vi "probe_freq_sweep.vi"() -> ()   [LabVIEW 2017]
doc: "Use this template to build a simple state machine design pattern. Each state executes code and determines which state to transition to."
uses:
  controls/State.ctl
  <userlib>/niRF/niQuickSyn/Core/Properties/Ref Output/PropertyType.ctl
  <userlib>/niRF/niQuickSyn/Core/Properties/Reference Source/PropertyType.ctl
  <instrlib>/niRFSA/niRFSA.llb/niRFSA Acquisition Types.ctl
  <userlib>/niRF/niQuickSyn/Core/Properties/RF Output/PropertyType.ctl
  <userlib>/niRF/niQuickSyn/Core/Typedefs/Session Handle.ctl
  <userlib>/niRF/niQuickSyn/Core/QuickSyn.lvclass
  <vilib>/Utility/error.llb/DialogType.ctl
  <vilib>/Analysis/1siggen.llb/Ramp Pattern by Samples.vi
  <instrlib>/niRFSA/niRFSA.llb/niRFSA Configure Spectrum Frequency Start Stop.vi
  <instrlib>/niRFSA/niRFSA.llb/niRFSA Read Power Spectrum (DBL).vi
  <userlib>/niRF/niQuickSyn/QuickSyn API.lvlib
  <userlib>/niRF/niQuickSyn/Core/Properties/Ref Output/Ref Output.lvclass
  <userlib>/niRF/niQuickSyn/Core/Properties/Reference Source/Ref Source.lvclass
  <userlib>/niRF/niQuickSyn/Core/Properties/RF Output/RF Output.lvclass
  <vilib>/Analysis/NI_AALBase.lvlib
panel:
  in  "Averaging":i32=1000 min=1 max=3201 step=1
  out "error out":errorcluster
  out "QuickSyn Resource Name Out":refnum<visa-resource-name>
  out "RFSA Resource Name Out":refnum<k15>
  in  "error in (no error)":errorcluster
  in  "Folder":string="Test"
  in  "Resolution Bandwidth RFSA":dbl=100000.0 caption="Resolution Bandwidth (Hz)" min=1.0 max=25000000.0 step=1.0 format="%#_6p"
  in  "Reference Power RFSA":dbl=1.0 caption="Reference Level (dBm)" min=-25.0 max=13.0 step=0.1
  in  "Stop Frequncy RFSA":dbl=2000000000.0 caption="Stop Frequncy (Hz)" min=500000000.0 max=20000000000.0 format="%#_6p"
  in  "Start Frequency RFSA":dbl=1000000000.0 caption="Start Frequency (Hz)" min=500000000.0 max=20000000000.0 format="%#_6p"
  in  "Output Power QuickSyn":dbl=1.0 caption="Output Power (dBm)" min=-25.0 max=13.0 step=0.1
  in  "Number of Points QuickSyn":i32=1000 caption="Number of Points" min=2 max=3201 step=1
  in  "Stop Frequncy QuickSyn":dbl=2000000000.0 caption="Stop Frequncy (Hz)" min=500000000.0 max=20000000000.0 format="%#_6p"
  in  "Start Frequency QuickSyn":dbl=1000000000.0 caption="Start Frequency (Hz)" min=500000000.0 max=20000000000.0 format="%#_6p"
  in  "QuickSyn Resource Name In":refnum<visa-resource-name>="COM5"
  in  "RFSA Resource Name In":refnum<k15>="RFSA_5665" caption="RFSA Resource Name"
  in  "Exit Button":bool
  out "Status":string="Shutting down...Sweeping field to zero..."
  out "Cursor":cluster{"x":dbl, "y":dbl} {"x" format="%.2f"; "y" format="%.5f"}
  out "SpectrumGraph":cluster{"Field":dbl[], "Signal":dbl[]}(graph)
  in  "Start Button":bool
  in  "Stop Button":bool
  # "Signal Generator"
  # "RF Spectrum Analyzer"
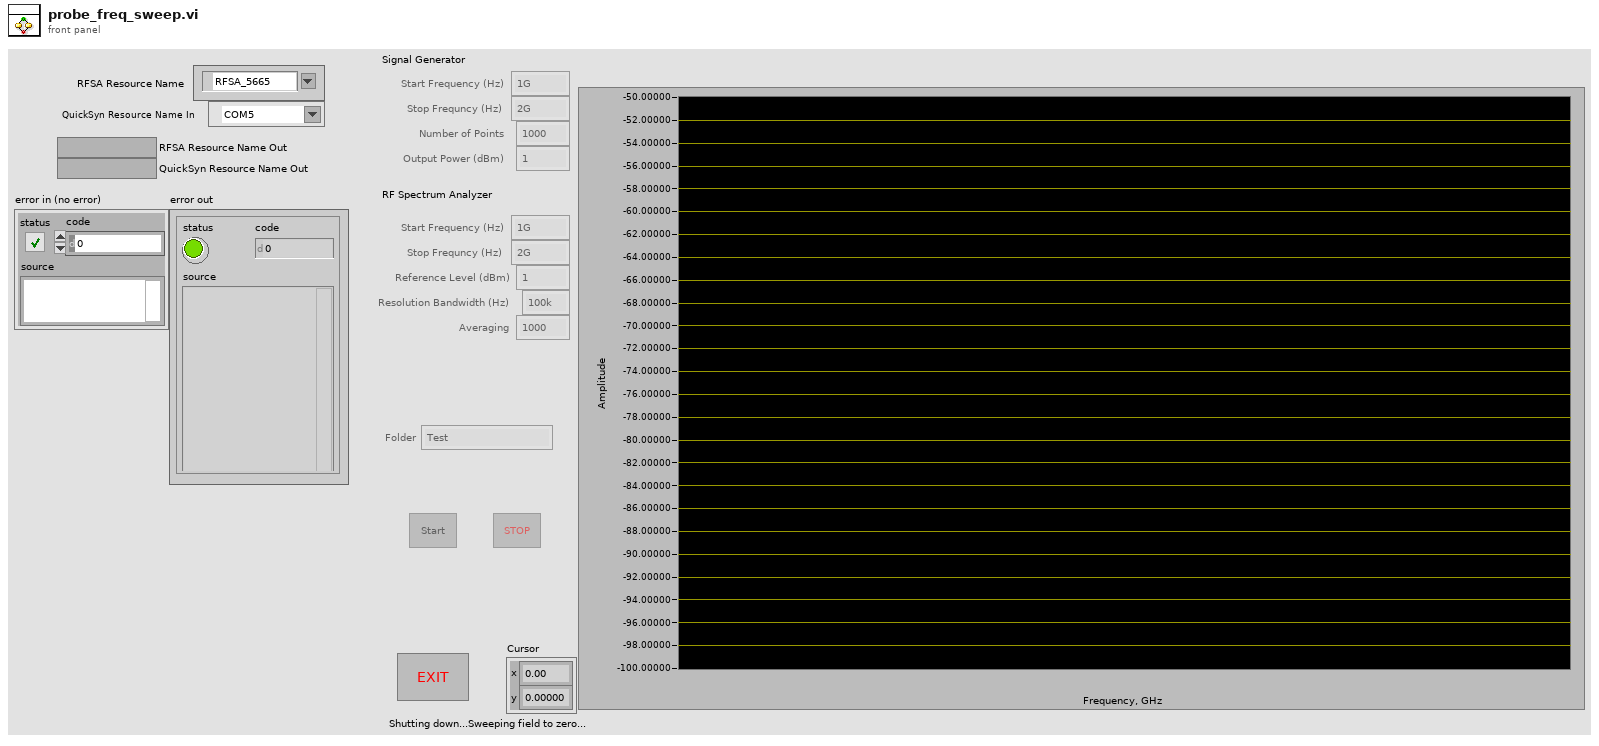
[diagram p1: front panel]
types:
  T1 = typedef "State.ctl" = enum16{"Init", "Idle", "Starting Meas", "Running", "Stopping Meas", "Shutting down"}
  T2 = typedef "QuickSyn API.lvlib/Ref Source.lvclass/PropertyType.ctl" = enum16{"Internal", "External"}
  T3 = typedef "QuickSyn API.lvlib/Ref Output.lvclass/PropertyType.ctl" = bool
  T4 = typedef "QuickSyn API.lvlib/RF Output.lvclass/PropertyType.ctl" = bool
  T5 = typedef "QuickSyn API.lvlib/QuickSyn.lvclass/Session Handle.ctl" = refnum<data-value>
  T6 = typedef "niRFSA Acquisition Types.ctl" = i32
  T7 = typedef "DialogType.ctl" = u16
  T8 = typedef "LVPoint32TypeDef.ctl" = cluster{"Horizontal":i32, "Vertical":i32}
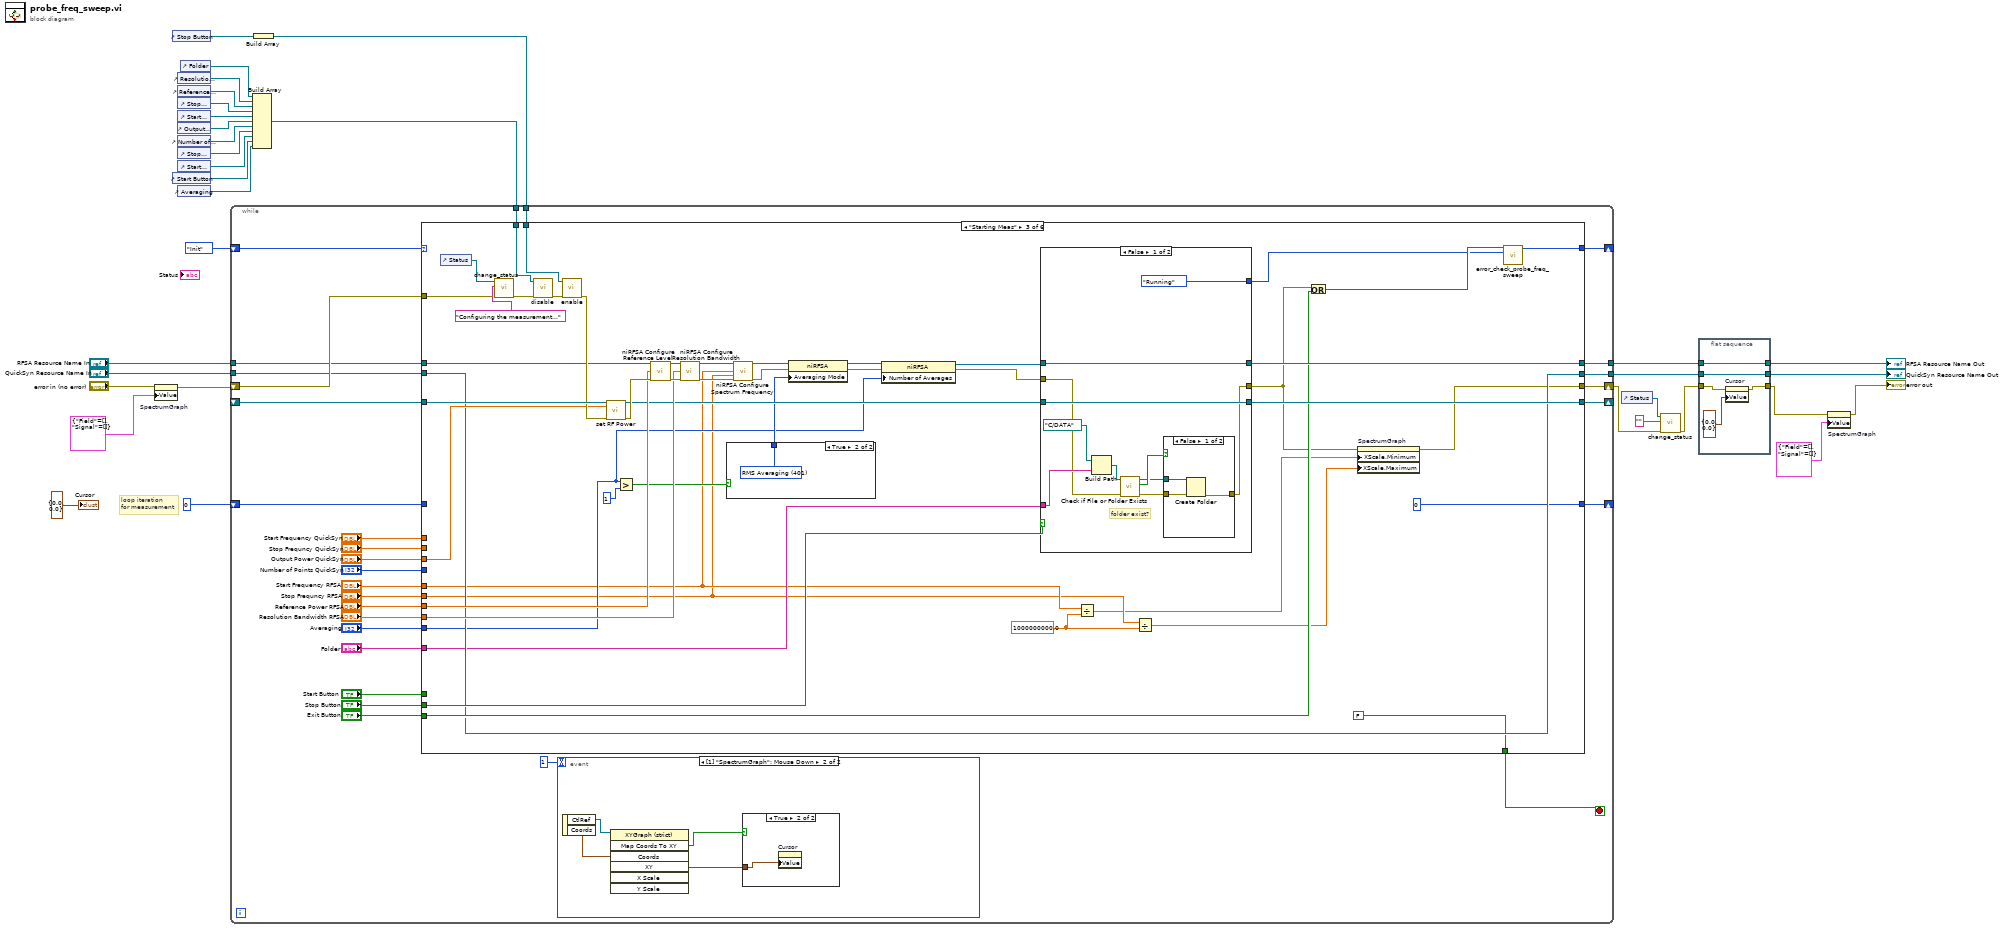
[diagram p0: block diagram]
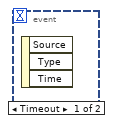
[diagram p2: hidden frame]
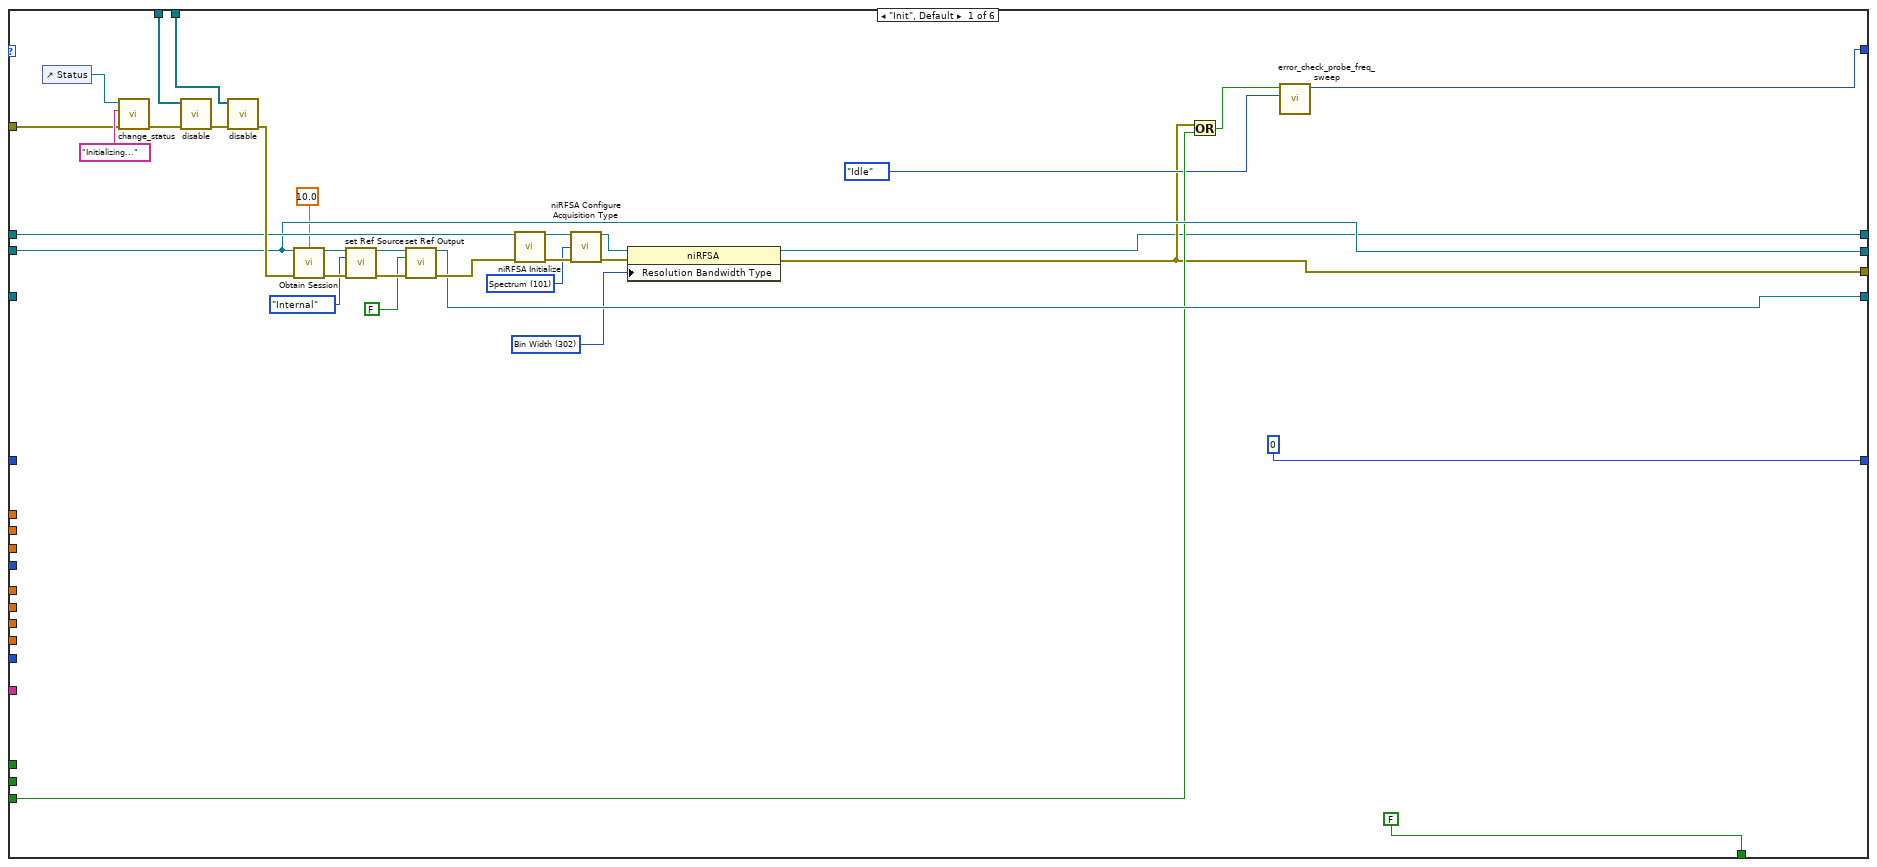
[diagram p4: hidden frame]
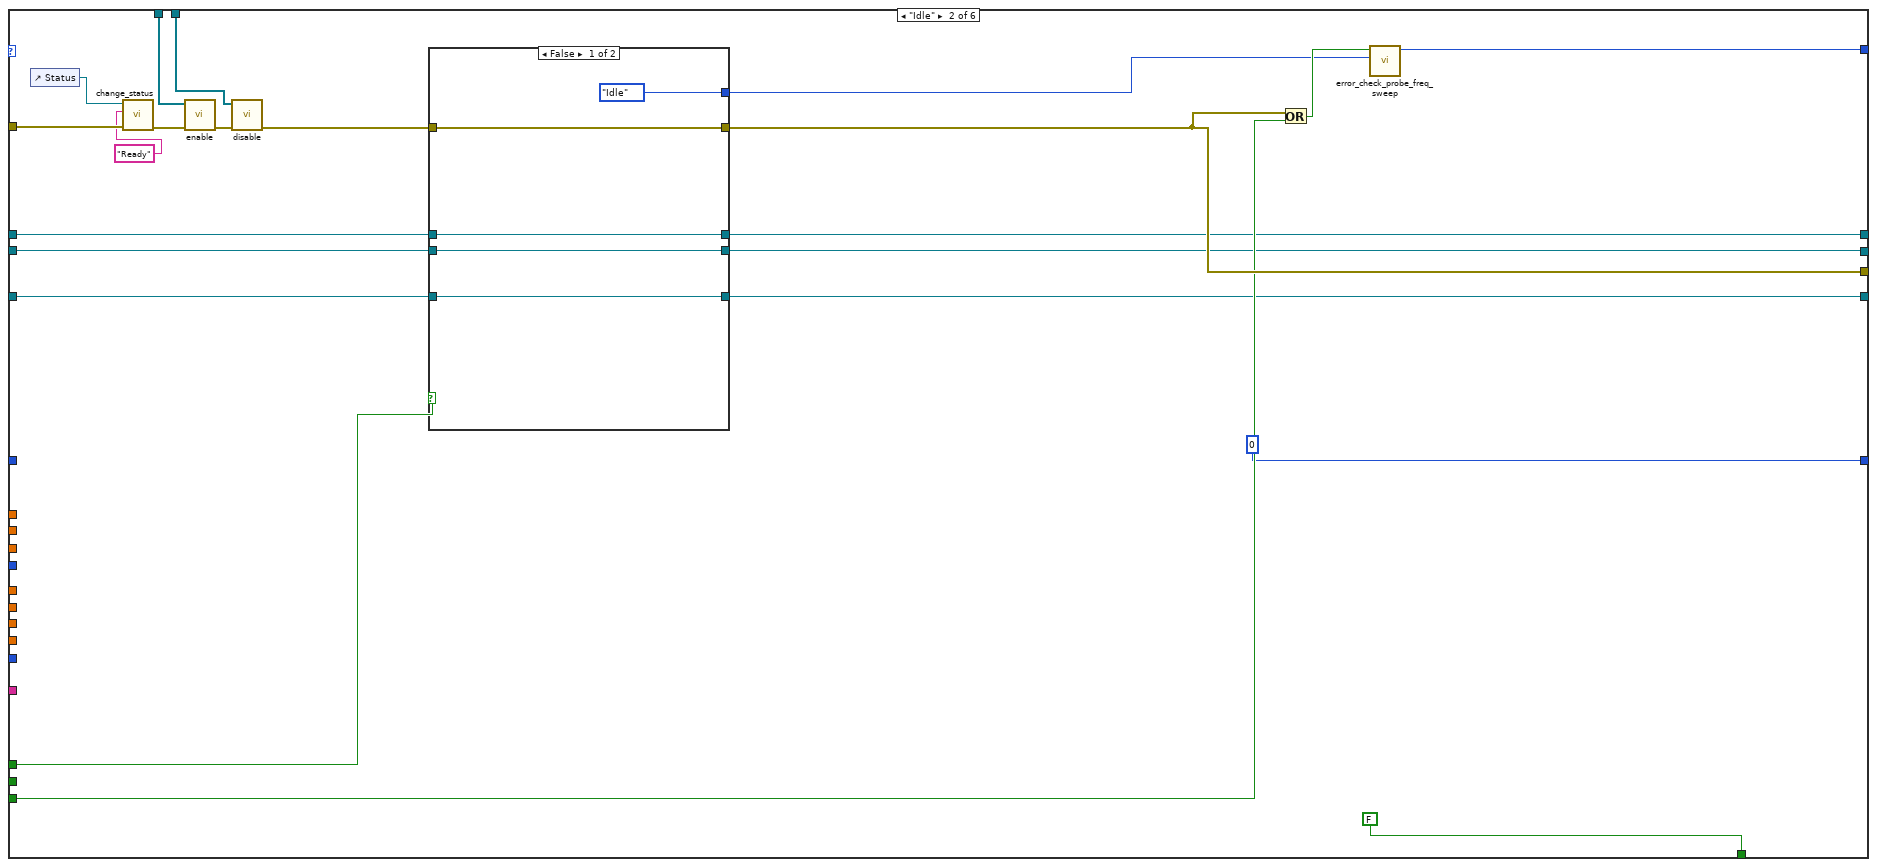
[diagram p5: hidden frame]
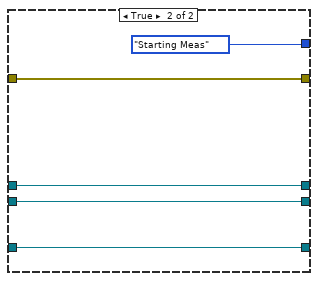
[diagram p6: hidden frame]
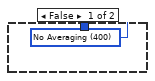
[diagram p7: hidden frame]
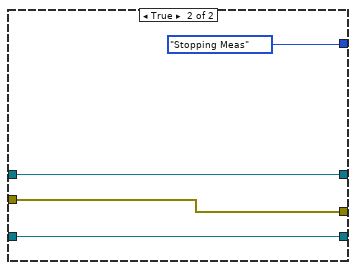
[diagram p9: hidden frame]
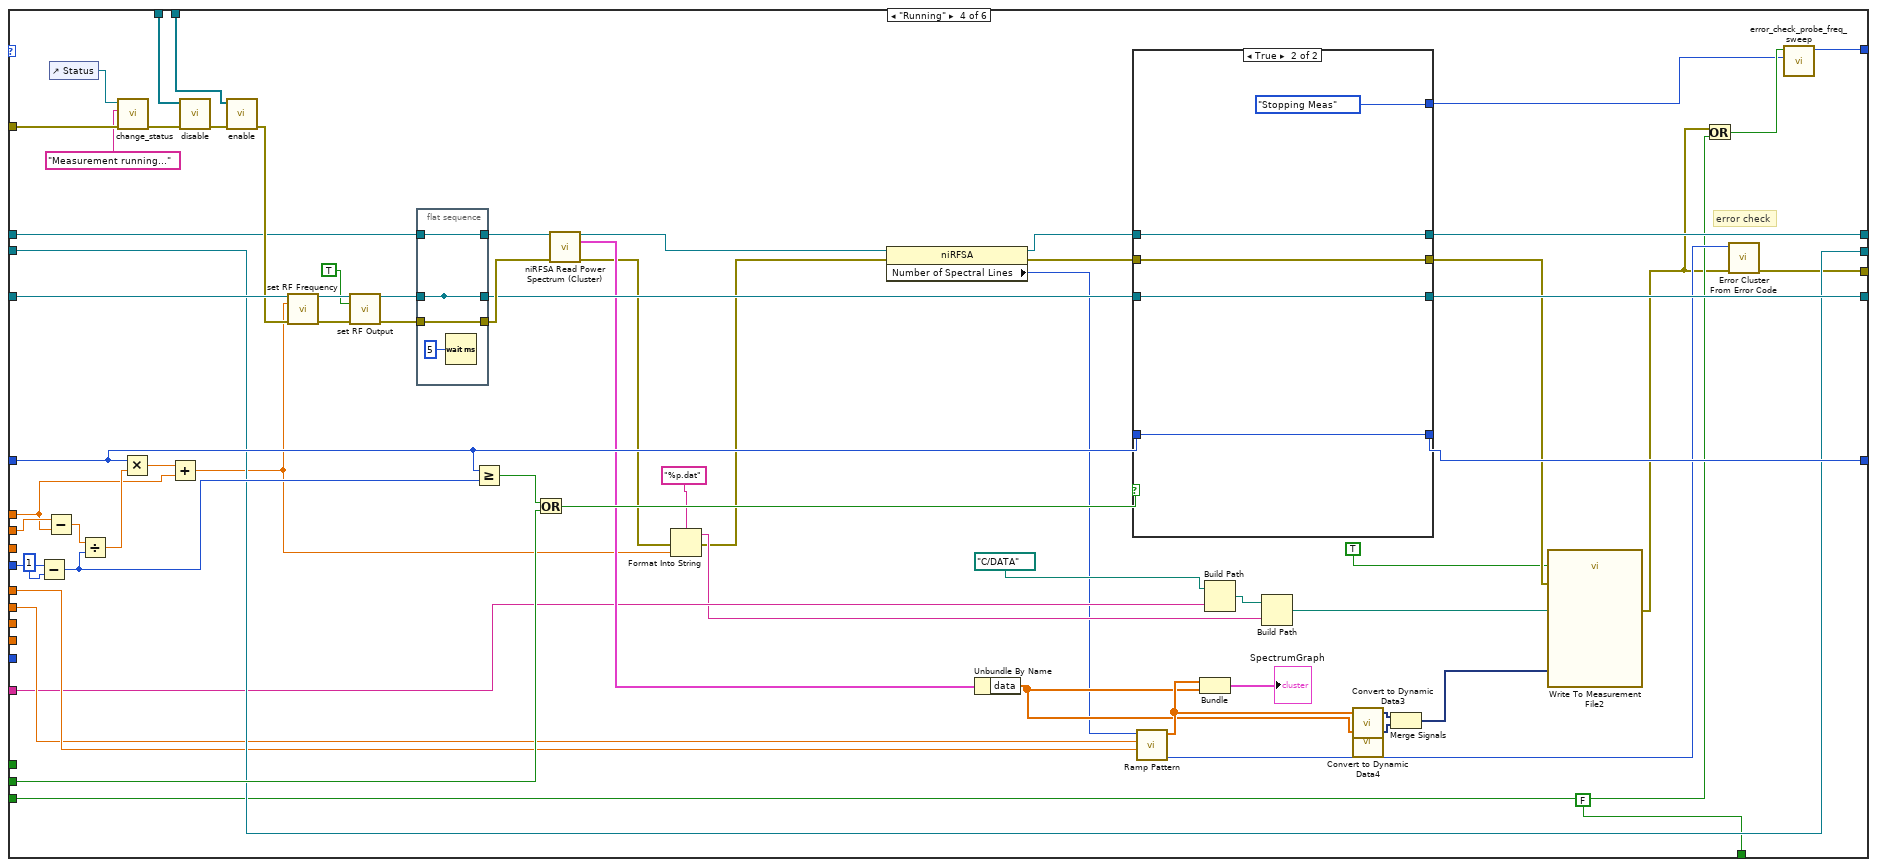
[diagram p10: hidden frame]
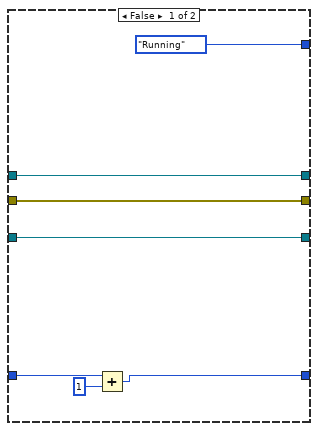
[diagram p11: hidden frame]
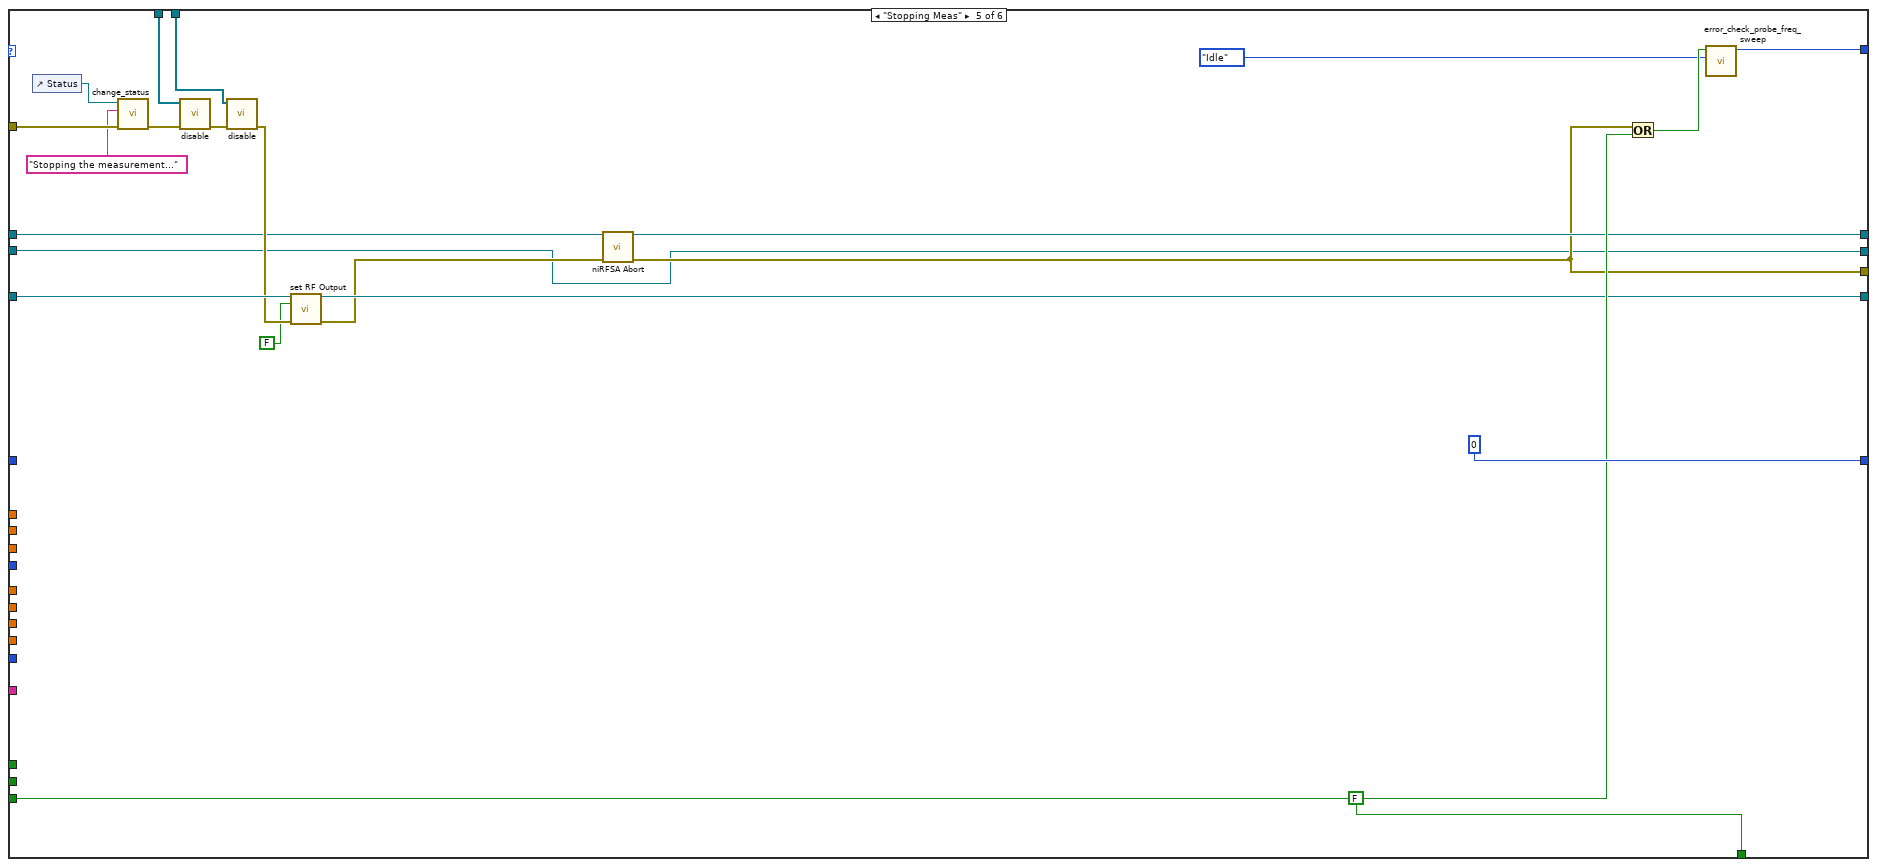
[diagram p12: hidden frame]
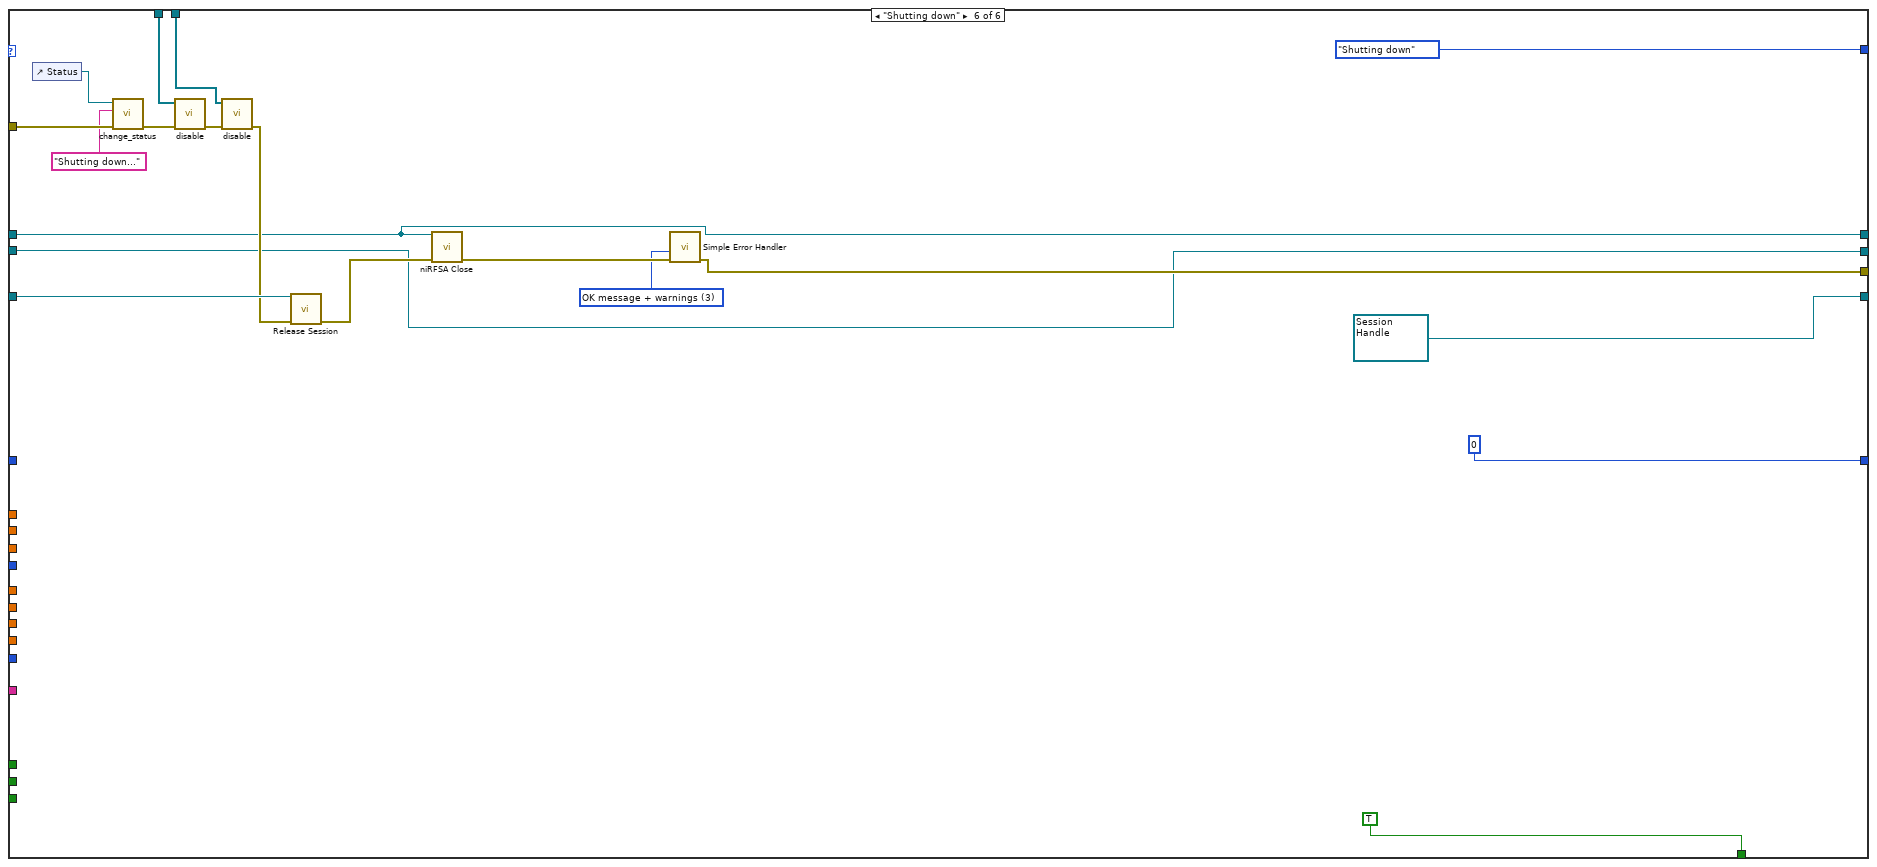
[diagram p13: hidden frame]
diagram:
  # "loop iteration\nfor measurement"
  n1 = property on="SpectrumGraph" class="XYGraph (strict)"(error in="error in (no error)", "Value"=cluster{"Field":dbl[], "Signal":dbl[]} {"Field"=[], "Signal"=[]} ("SpectrumGraph")) -> (error out=w18:errorcluster)  [unwired: 1 in, 1 out]
  n2 = control-ref of="Stop Button"() -> (w22:refnum<vi>)
  n3 = control-ref of="Start Button"() -> (w23:refnum<vi>)
  n4 = control-ref of="Resolution Bandwidth RFSA"() -> (w14:refnum<vi>)
  n5 = control-ref of="Reference Power RFSA"() -> (w15:refnum<vi>)
  n6 = control-ref of="Stop Frequncy RFSA"() -> (w30:refnum<vi>)
  n7 = control-ref of="Start Frequency RFSA"() -> (w29:refnum<vi>)
  n8 = control-ref of="Output Power QuickSyn"() -> (w28:refnum<vi>)
  n9 = control-ref of="Number of Points QuickSyn"() -> (w27:refnum<vi>)
  n10 = control-ref of="Stop Frequncy QuickSyn"() -> (w26:refnum<vi>)
  n11 = control-ref of="Start Frequency QuickSyn"() -> (w25:refnum<vi>)
  n12 = control-ref of="Averaging"() -> (w1:refnum<vi>)
  n13 = control-ref of="Folder"() -> (w13:refnum<vi>)
  n14 = Build Array(w13, w14, w15, w30, w29, w28, w27, w26, w25, w23, w1) -> (w24:refnum<vi>[])
  n15 = Build Array(w22) -> (w21:refnum<vi>[])
  n16 = while {
    tunnel: "RFSA Resource Name In" -> [w60]
    tunnel: "QuickSyn Resource Name In" -> [w59]
    tunnel: w24 -> [w58]
    tunnel: w21 -> [w57]
    tunnel: [w44] -> w9
    tunnel: [w43] -> w7
    shift-right: [w42] -> _
    shift-left: State."Init" ("States") -> [w62]
    shift-right: [w41] -> w12
    shift-left: w18 -> [w61]
    shift-right: [w40] -> _
    shift-left: _ -> [w39]
    shift-right: [w37] -> _
    shift-left: 0 -> [w38]
    stop <- w35 stop-if-true
    n17 = case shown="\"Starting Meas\"" w62 {
      tunnel: w61 -> [w99 w120 w176 w266 w300 w323]
      tunnel: w60 -> [w86 w108 w170 w247 w287 w307]
      tunnel: w59 -> [w80 w107 w154 w230 w283 w306]
      tunnel: w58 -> [w96 w119 w174 w264 w304 w322]
      tunnel: w57 -> [w95 w118 w175 w265 w303 w321]
      tunnel: "Start Frequency QuickSyn" -> [_ _ _ w248 _ _]
      tunnel: "Stop Frequncy QuickSyn" -> [_ _ _ w259 _ _]
      tunnel: "Output Power QuickSyn" -> [_ _ w171 _ _ _]
      tunnel: "Number of Points QuickSyn" -> [_ _ _ w258 _ _]
      tunnel: "Start Frequency RFSA" -> [_ _ w137 w228 _ _]
      tunnel: "Stop Frequncy RFSA" -> [_ _ w136 w227 _ _]
      tunnel: "Reference Power RFSA" -> [_ _ w166 _ _ _]
      tunnel: "Resolution Bandwidth RFSA" -> [_ _ w165 _ _ _]
      tunnel: "Folder" -> [_ _ w151 w216 _ _]
      tunnel: "Start Button" -> [_ w115 _ _ _ _]
      tunnel: "Stop Button" -> [_ _ w162 w239 _ _]
      tunnel: "Exit Button" -> [w79 w111 w156 w223 w290 _]
      tunnel: [w81 w103 w159 w231 w289 T5 refnum ("Session Handle out")] -> w40
      tunnel: [w69 w105 w160 w232 w286 w307] -> w44
      tunnel: [w80 w104 w154 w230 w283 w306] -> w43
      tunnel: [w71 w112 w148 w225 w284 w308] -> w41
      tunnel: [w76 w109 w157 w235 w293 State."Shutting down" ("f out")] -> w42
      tunnel: w39 -> [_ w106 w173 w255 w297 w316]
      tunnel: w38 -> [_ _ _ w237 _ _]
      tunnel: [0 0 0 w236 0 0] -> w37
      tunnel: [FALSE FALSE FALSE FALSE FALSE TRUE] -> w35
      tunnel: "Averaging" -> [_ _ w138 _ _ _]
      frame "Init", Default {
        w68 = 302 items=["3dB"=300, "6dB"=301, "Bin Width"=302, "ENBW"=303] ("Acquisition:Spectrum:Resolution Bandwidth Type")
        w82 = T6 101 items=["IQ"=100, "Spectrum"=101] ("acquisition type")
        n18 = control-ref of="Status"() -> (w97:refnum<vi>)
        n19 = call "change_status.vi"("error in (no error)"=w99, "String"="Initializing...", "String in"=w97) -> ("error out"=w98:errorcluster)  [unwired: 8 in]
        n20 = call "disable.vi"("error in (no error)"=w98, "Array"=w96) -> ("error out"=w94:errorcluster)  [unwired: 9 in]
        n21 = call "disable.vi"("error in (no error)"=w94, "Array"=w95) -> ("error out"=w93:errorcluster)  [unwired: 9 in]
        n22 = call <userlib>:"Obtain Session.vi"("VISA resource name"=w80, "Serial Timeout"=10.0, "error in (no error)"=w93) -> ("Session Handle"=w90:T5, "error out"=w92:errorcluster)  [unwired: 11 in]
        n23 = call <userlib>:"set Ref Source.vi"("Session Handle in"=w90, "Ref Source (Internal)"=PropertyType."Internal", "error in (no error)"=w92) -> ("Session Handle out"=w89:T5, "error out"=w91:errorcluster)  [unwired: 11 in]
        n24 = call <userlib>:"set Ref Output.vi"("Session Handle in"=w89, "Ref Output (False)"=T3 FALSE, "error in (no error)"=w91) -> ("Session Handle out"=w81:T5, "error out"=w84:errorcluster)  [unwired: 11 in]
        n25 = call <instrlib>:"niRFSA Initialize.vi"("resource name"=w86, "error in"=w84) -> ("instrument handle out"=w85:refnum<k15>, "error out"=w83:errorcluster)  [unwired: 12 in]
        n26 = call <instrlib>:"niRFSA Configure Acquisition Type.vi"("instrument handle"=w85, "acquisition type"=w82, "error in"=w83) -> ("instrument handle out"=w70:refnum<k15>, "error out"=w72:errorcluster)  [unwired: 11 in]
        n27 = property class="niRFSA"(reference=w70, error in=w72, "Resolution Bandwidth Type"=w68) -> (reference out=w69:refnum<k15>, error out=w71:errorcluster)
        n28 = Or(x=w71, y=w79) -> (x .or. y?=w78:bool)
        n29 = call "error_check_probe_freq_sweep.vi"("f in"=State."Idle" ("f"), "Boolean"=w78) -> ("f out"=w76:T1)  [unwired: 9 in]
      }
      frame "Idle" {
        n30 = control-ref of="Status"() -> (w116:refnum<vi>)
        n31 = call "change_status.vi"("error in (no error)"=w120, "String"="Ready", "String in"=w116) -> ("error out"=w121:errorcluster)  [unwired: 8 in]
        n32 = call "enable.vi"("error in (no error)"=w121, "Array"=w119) -> ("error out"=w122:errorcluster)  [unwired: 9 in]
        n33 = call "disable.vi"("error in (no error)"=w122, "Array"=w118) -> ("error out"=w114:errorcluster)  [unwired: 9 in]
        n34 = case shown="False" w115 {
          tunnel: w114 -> [w126 w131]
          tunnel: [State."Idle" ("States") State."Starting Meas" ("States")] -> w110
          tunnel: [w126 w131] -> w112
          tunnel: w108 -> [w125 w130]
          tunnel: w107 -> [w124 w129]
          tunnel: [w125 w130] -> w105
          tunnel: [w124 w129] -> w104
          tunnel: w106 -> [w123 w128]
          tunnel: [w123 w128] -> w103
          frame False {
          }
          frame True {
          }
        }
        n35 = Or(x=w112, y=w111) -> (x .or. y?=w113:bool)
        n36 = call "error_check_probe_freq_sweep.vi"("f in"=w110, "Boolean"=w113) -> ("f out"=w109:T1)  [unwired: 9 in]
      }
      frame "Starting Meas" {
        w135 = 1000000000.0 ("y")
        n37 = control-ref of="Status"() -> (w153:refnum<vi>)
        n38 = call "change_status.vi"("error in (no error)"=w176, "String"="Configuring the measurement...", "String in"=w153) -> ("error out"=w178:errorcluster)  [unwired: 8 in]
        n39 = call "disable.vi"("error in (no error)"=w178, "Array"=w174) -> ("error out"=w179:errorcluster)  [unwired: 9 in]
        n40 = call "enable.vi"("error in (no error)"=w179, "Array"=w175) -> ("error out"=w172:errorcluster)  [unwired: 9 in]
        n41 = call <userlib>:"set RF Power.vi"("Session Handle in"=w173, "RF Power, dB (0)"=w171, "error in (no error)"=w172) -> ("Session Handle out"=w161:T5, "error out"=w168:errorcluster)  [unwired: 11 in]
        n42 = Greater?(x=w138, y=1) -> (0:w144:bool)
        n43 = call <instrlib>:"niRFSA Configure Reference Level.vi"("instrument handle"=w170, "reference level (dBm)"=w166, "error in"=w168) -> ("instrument handle out"=w169:refnum<k15>, "error out"=w167:errorcluster)  [unwired: 11 in]
        n44 = call <instrlib>:"niRFSA Configure Resolution Bandwidth.vi"("instrument handle"=w169, "resolution bandwidth (Hz)"=w165, "error in"=w167) -> ("instrument handle out"=w164:refnum<k15>, "error out"=w163:errorcluster)  [unwired: 11 in]
        n45 = case shown="True" w144 {
          tunnel: [w180 w181] -> w143
          frame False {
            w180 = 400 items=["No Averaging"=400, "RMS Averaging"=401, "Vector Averaging"=402, "Peak Hold Averaging"=403, "Min Hold Averaging"=404, "Scalar Averaging"=405, "Log Averaging"=406] ("Acquisition:Spectrum:Averaging Mode")
          }
          frame True {
            w181 = 401 items=["No Averaging"=400, "RMS Averaging"=401, "Vector Averaging"=402, "Peak Hold Averaging"=403, "Min Hold Averaging"=404, "Scalar Averaging"=405, "Log Averaging"=406] ("Acquisition:Spectrum:Averaging Mode")
          }
        }
        n46 = call-poly <instrlib>:"niRFSA Configure Spectrum Frequency.vi"("instrument handle"=w164, "start frequency"=w137, "stop frequency"=w136, "error in"=w163) -> ("instrument handle out"=w147:refnum<k15>, "error out"=w146:errorcluster)  [unwired: 10 in]
        n47 = property class="niRFSA"(reference=w147, error in=w146, "Averaging Mode"=w143) -> (reference out=w142:refnum<k15>, error out=w140:errorcluster)
        n48 = property class="niRFSA"(reference=w142, error in=w140, "Number of Averages"=w138) -> (reference out=w141:refnum<k15>, error out=w139:errorcluster)
        n49 = case shown="False" w162 {
          tunnel: [State."Running" ("States") State."Stopping Meas" ("States")] -> w155
          tunnel: w139 -> [w187 w198]
          tunnel: w141 -> [w191 w199]
          tunnel: w161 -> [w190 w197]
          tunnel: [w191 w199] -> w160
          tunnel: [w183 w198] -> w149
          tunnel: [w190 w197] -> w159
          tunnel: w151 -> [w188 _]
          frame False {
            # "folder exist?"
            n50 = Build Path(base path=path "C:/DATA" ("file path (use dialog)"), name or relative path=w188) -> (appended path=w186:path)
            n51 = call <vilib>:"Check if File or Folder Exists.vi"("error in (no error)"=w187, "path"=w186) -> ("error out"=w184:errorcluster, "file or folder exists?"=w185:bool, "dup path"=w182:path)  [unwired: 7 in]
            n52 = case shown="False" w185 {
              tunnel: w184 -> [w195 w196]
              tunnel: [w194 w196] -> w183
              tunnel: w182 -> [w193 _]
              frame False {
                n53 = Create Folder(path (use dialog)=w193, error in=w195) -> (error out=w194:errorcluster)  [unwired: 1 in, 2 out]
              }
              frame True {
                # "create folder"
              }
            }
          }
          frame True {
          }
        }
        n54 = Divide(x=w137, y=w135) -> (x/y=w134:dbl)
        n55 = Divide(x=w136, y=w135) -> (x/y=w133:dbl)
        n56 = Or(x=w149, y=w156) -> (x .or. y?=w158:bool)
        n57 = property on="SpectrumGraph" class="XYGraph (strict)"(error in=w149, "XScale.Minimum"=w134, "XScale.Maximum"=w133) -> (error out=w148:errorcluster)  [unwired: 1 in, 1 out]
        n58 = call "error_check_probe_freq_sweep.vi"("f in"=w155, "Boolean"=w158) -> ("f out"=w157:T1)  [unwired: 9 in]
      }
      frame "Running" {
        # "error check"
        n59 = Subtract(x=w258, y=1) -> (x-y=w241:i32)
        n60 = Subtract(x=w259, y=w248) -> (x-y=w256:dbl)
        n61 = control-ref of="Status"() -> (w260:refnum<vi>)
        n62 = Divide(x=w256, y=w241) -> (x/y=w250:dbl)
        n63 = call "change_status.vi"("error in (no error)"=w266, "String"="Measurement running...", "String in"=w260) -> ("error out"=w263:errorcluster)  [unwired: 8 in]
        n64 = Multiply(x=w237, y=w250) -> (x*y=w249:dbl)
        n65 = Add(x=w249, y=w248) -> (x+y=w211:dbl)
        n66 = call "disable.vi"("error in (no error)"=w263, "Array"=w264) -> ("error out"=w262:errorcluster)  [unwired: 9 in]
        n67 = call "enable.vi"("error in (no error)"=w262, "Array"=w265) -> ("error out"=w253:errorcluster)  [unwired: 9 in]
        n68 = call <userlib>:"set RF Frequency.vi"("Session Handle in"=w255, "RF Frequency, Hz (200M)"=w211, "error in (no error)"=w253) -> ("Session Handle out"=w254:T5, "error out"=w252:errorcluster)  [unwired: 11 in]
        n69 = call <userlib>:"set RF Output.vi"("Session Handle in"=w254, "RF Output (False)"=T4 TRUE, "error in (no error)"=w252) -> ("Session Handle out"=w245:T5, "error out"=w244:errorcluster)  [unwired: 11 in]
        n70 = flat-sequence {
          tunnel: w247 -> [w282]
          tunnel: [w282] -> w246
          tunnel: [w279] -> _
          tunnel: w245 -> [w279]
          tunnel: [w281] -> w243
          tunnel: w244 -> [w281]
          tunnel: [w279] -> w242
          frame #0 {
            n71 = Wait (ms)(milliseconds to wait=u32 5) -> ()  [unwired: 1 out]
          }
        }
        n72 = Greater Or Equal?(x=w237, y=w241) -> (x >= y?=w240:bool)
        n73 = Or(x=w240, y=w239) -> (x .or. y?=w238:bool)
        n74 = call-poly <instrlib>:"niRFSA Read Power Spectrum (Cluster).vi"("instrument handle"=w246, "error in"=w243) -> ("instrument handle out"=w202:refnum<k15>, "power spectrum"=w229:cluster{"f0":dbl, "df":dbl, "data":dbl[]}, "error out"=w214:errorcluster)  [unwired: 11 in]
        n75 = Format Into String(format string="%p.dat", error in=w214, w211) -> (resulting string=w213:string, error out=w205:errorcluster)  [unwired: 1 in]
        n76 = property class="niRFSA"(reference=w202, error in=w205) -> (reference out=w201:refnum<k15>, error out=w204:errorcluster, "Number of Spectral Lines"=w203:i32)
        n77 = Unbundle By Name(w229) -> ("data"=w219:dbl[])
        n78 = case shown="True" w238 {
          tunnel: [State."Running" ("States") State."Stopping Meas" ("States")] -> w233
          tunnel: w204 -> [w271 w276]
          tunnel: w201 -> [w272 w277]
          tunnel: w242 -> [w270 w275]
          tunnel: [w272 w277] -> w232
          tunnel: [w271 w276] -> w209
          tunnel: [w270 w275] -> w231
          tunnel: w237 -> [w269 w274]
          tunnel: [w267 w274] -> w236
          frame False {
            n79 = Add(x=w269, y=1) -> (x+y=w267:i32)
          }
          frame True {
          }
        }
        n80 = call-poly <vilib>:"Ramp Pattern.vi"("start"=w228, "end"=w227, "samples"=w203) -> ("error"=w224:i32, "Ramp Pattern"=w222:dbl[])  [unwired: 7 in]
        n81 = Bundle("Ramp Pattern"=w222, "data"=w219) -> (→"SpectrumGraph":cluster{"Ramp Pattern":dbl[], "data":dbl[]})  [unwired: 1 in]
        n82 = Build Path(base path=path "C:/DATA" ("Filename"), name or relative path=w216) -> (appended path=w215:path)
        n83 = Build Path(base path=w215, name or relative path=w213) -> (appended path=w212:path)
        n84 = call "Convert to Dynamic Data3"("Array"=w222) -> ("Dynamic Data Type"=w221:dynamicdata)  [unwired: 3 in]
        n85 = call "Convert to Dynamic Data4"("Array"=w219) -> ("Dynamic Data Type"=w218:dynamicdata)  [unwired: 3 in]
        n86 = Merge Signals(w221, w218) -> (w220:dynamicdata)
        n87 = call "Write To Measurement File2"("Signals"=w220, "Reset"=TRUE, "error in (no error)"=w209, "Filename"=w212) -> ("error out"=w208:errorcluster)  [unwired: 13 in, 2 out]
        n88 = Or(x=w208, y=w223) -> (x .or. y?=w234:bool)
        n89 = call <vilib>:"Error Cluster From Error Code.vi"("error in (no error)"=w208, "error code (0)"=w224) -> ("error out"=w225:errorcluster)  [unwired: 7 in]
        n90 = call "error_check_probe_freq_sweep.vi"("f in"=w233, "Boolean"=w234) -> ("f out"=w235:T1)  [unwired: 9 in]
      }
      frame "Stopping Meas" {
        n91 = control-ref of="Status"() -> (w298:refnum<vi>)
        n92 = call "change_status.vi"("error in (no error)"=w300, "String"="Stopping the measurement...", "String in"=w298) -> ("error out"=w302:errorcluster)  [unwired: 8 in]
        n93 = call "disable.vi"("error in (no error)"=w302, "Array"=w304) -> ("error out"=w301:errorcluster)  [unwired: 9 in]
        n94 = call "disable.vi"("error in (no error)"=w301, "Array"=w303) -> ("error out"=w296:errorcluster)  [unwired: 9 in]
        n95 = call <userlib>:"set RF Output.vi"("Session Handle in"=w297, "RF Output (False)"=T4 FALSE, "error in (no error)"=w296) -> ("Session Handle out"=w289:T5, "error out"=w285:errorcluster)  [unwired: 11 in]
        n96 = call <instrlib>:"niRFSA Abort.vi"("instrument handle"=w287, "error in"=w285) -> ("instrument handle out"=w286:refnum<k15>, "error out"=w284:errorcluster)  [unwired: 12 in]
        n97 = Or(x=w284, y=w290) -> (x .or. y?=w292:bool)
        n98 = call "error_check_probe_freq_sweep.vi"("f in"=State."Idle", "Boolean"=w292) -> ("f out"=w293:T1)  [unwired: 9 in]
      }
      frame "Shutting down" {
        w309 = T7 3 items=["no dialog", "OK message", "continue or stop message", "OK message + warnings", "continue/stop + warnings"] ("type of dialog (OK msg:1)")
        n99 = control-ref of="Status"() -> (w318:refnum<vi>)
        n100 = call "change_status.vi"("error in (no error)"=w323, "String"="Shutting down...", "String in"=w318) -> ("error out"=w320:errorcluster)  [unwired: 8 in]
        n101 = call "disable.vi"("error in (no error)"=w320, "Array"=w322) -> ("error out"=w319:errorcluster)  [unwired: 9 in]
        n102 = call "disable.vi"("error in (no error)"=w319, "Array"=w321) -> ("error out"=w315:errorcluster)  [unwired: 9 in]
        n103 = call <userlib>:"Release Session.vi"("Session Handle"=w316, "error in (no error)"=w315) -> ("error out"=w311:errorcluster)  [unwired: 13 in]
        n104 = call <instrlib>:"niRFSA Close.vi"("instrument handle"=w307, "error in"=w311) -> ("error out"=w310:errorcluster)  [unwired: 13 in]
        n105 = call <vilib>:"Simple Error Handler.vi"("type of dialog (OK msg:1)"=w309, "error in (no error)"=w310) -> ("error out"=w308:errorcluster)  [unwired: 3 in, 4 out]
      }
    }
    n106 = event shown="[1] \"SpectrumGraph\": Mouse Down" {
      selector: _ -> [_ _]
      dyn-events: _ -> [_ _]
      timeout: 1 -> [_ _]
      event Timeout {
        n107 = event-data() -> ()  [unwired: 1 in, 3 out]
      }
      event "SpectrumGraph": Mouse Down {
        n108 = event-data() -> ("CtlRef"=w66:refnum<vi>, "Coords"=w65:T8)  [unwired: 1 in]
        n109 = invoke class="XYGraph (strict)" method="Map Coords To XY"(reference=w66, "Coords"=w65) -> ("Map Coords To XY"=w64:bool, "XY"=w63:cluster{"X":dbl, "Y":dbl})  [unwired: 5 in, 5 out]
        n110 = case shown="True" w64 {
          tunnel: w63 -> [_ w67]
          frame False {
          }
          frame True {
            n111 = property on="Cursor" class="Clust (strict)"("Value"=w67) -> ()  [unwired: 2 in, 2 out]
          }
        }
      }
    }
  }
  n112 = control-ref of="Status"() -> (w11:refnum<vi>)
  n113 = call "change_status.vi"("error in (no error)"=w12, "String"="", "String in"=w11) -> ("error out"=w5:errorcluster)  [unwired: 8 in]
  n114 = flat-sequence {
    tunnel: w9 -> [w328]
    tunnel: [w328] -> w8
    tunnel: [w327] -> w6
    tunnel: w7 -> [w327]
    tunnel: w5 -> [w326]
    tunnel: [w325] -> w3
    frame #0 {
      n115 = property on="Cursor" class="Clust (strict)"(error in=w326, "Value"=cluster{"x":dbl, "y":dbl} {"x"=0.0, "y"=0.0} ("Cursor")) -> (error out=w325:errorcluster)  [unwired: 1 in, 1 out]
    }
  }
  n116 = property on="SpectrumGraph" class="XYGraph (strict)"(error in=w3, "Value"=cluster{"Field":dbl[], "Signal":dbl[]} {"Field"=[], "Signal"=[]} ("SpectrumGraph")) -> (error out=→"error out":errorcluster)  [unwired: 1 in, 1 out]
  "Cursor" <- cluster{"x":dbl, "y":dbl} {"x"=0.0, "y"=0.0} ("Cursor")
  "RFSA Resource Name Out" <- w8
  "QuickSyn Resource Name Out" <- w6
